vi "CPP-BLInterpolateTI.vi"() -> (0 "New Values In":string[][](array[string]), 1 "New Chs In":string[](array[string]))   [LabVIEW 2021]
uses:
  <vilib>/gmath/NI_Gmath.lvlib
  Data plotting/subVIs/Plot_Values_Global.vi
panel:
  in  "Requested TI height":dbl=254.0
  # "This VI receives  transposed plots of TI vs Z, and interpolates TI at the requested heights"
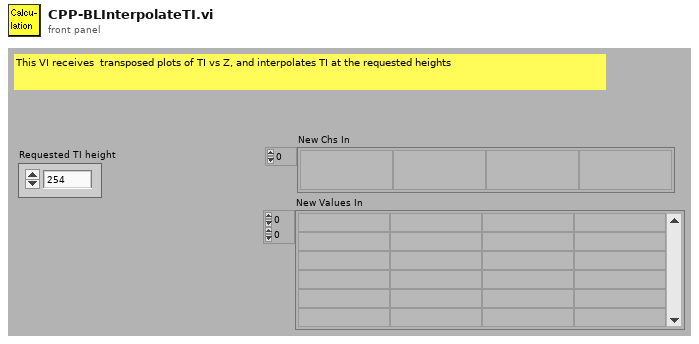
[diagram p1: front panel]
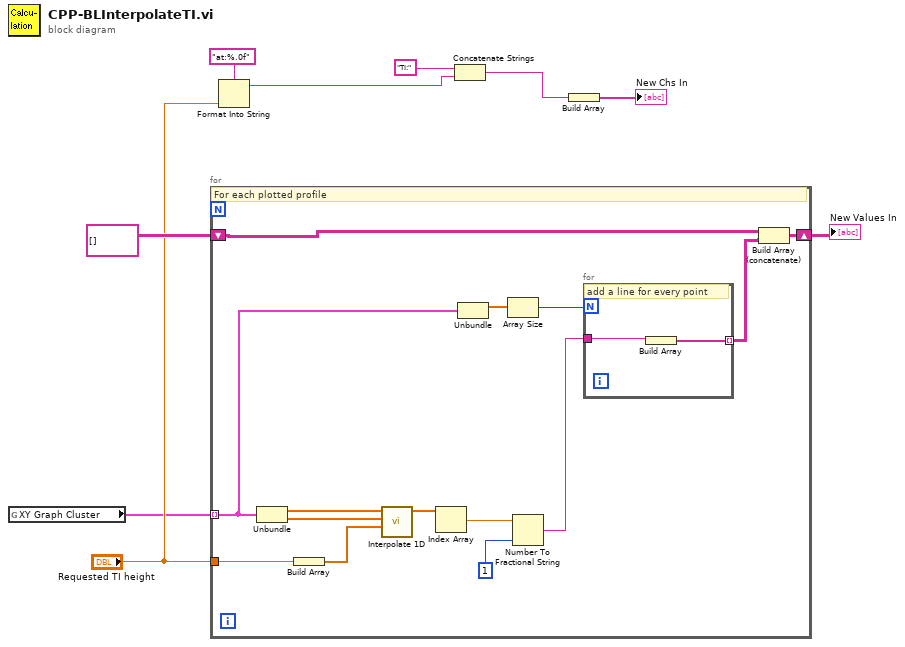
[diagram p0: block diagram]
diagram:
  n1 = global read "Plot_Values_Global.vi" "XY Graph Cluster"() -> (w1:cluster{dbl[], dbl[]}[])
  n2 = for {
    tunnel: w1 -> [w19] mode=indexing
    shift-right: [w23] -> w6
    shift-left: string[][] [] -> [w22]
    tunnel: "Requested TI height" -> [w15]
    # "For each plotted profile"
    n3 = Unbundle(w19) -> (w18:dbl[], w17:dbl[])
    n4 = Build Array(w15) -> (w16:dbl[])
    n5 = call <vilib>:"Interpolate 1D.vi"("xi"=w16, "X"=w17, "Y"=w18) -> ("yi"=w14:dbl[])  [unwired: 6 in, 2 out]
    n6 = Index Array(array=w14) -> (element=w13:dbl)  [unwired: 1 in]
    n7 = Unbundle(w19) -> (w20:dbl[])  [unwired: 1 out]
    n8 = Array Size(array=w20) -> (size(s)=w21:i32)
    n9 = Number To Fractional String(number=w13, precision (6)=i16 1) -> (F-format string=w12:string)  [unwired: 2 in]
    n10 = for {
      N: w21 -> [_]
      tunnel: w12 -> [w25]
      tunnel: [w24] -> w11 mode=indexing
      # "add a line for every point"
      n11 = Build Array(w25) -> (w24:string[])
    }
    n12 = Build Array (concatenate)(w22, w11) -> (w23:string[][])
  }
  "New Values In" <- w6
  n13 = Format Into String(format string="at:%.0f", "Requested TI height") -> (resulting string=w4:string)  [unwired: 2 in, 1 out]
  n14 = Concatenate Strings("TI:" ("string"), w4) -> (w8:string)
  n15 = Build Array(w8) -> (→"New Chs In":string[])
